vi "Read Waveform.vi"(8 "error in (no error)":errorcluster, 10 "Channel":T1, 11 "MSOX6004 in":refnum<class "MSOX6004.lvclass">) -> (0 "error out":errorcluster, 2 "Waveform":waveform(dbl)(graph), 3 "MSOX6004 out":refnum<class "MSOX6004.lvclass">)   [LabVIEW 2018, in "MSOX6004.lvlib" / "MSOX6004.lvclass"]
doc: "This Override method is used to initiate waveform acquisition. Select targeted channel at the 'Channel' control and output waveform data to the 'Waveform' indicator."
uses:
  MSOX6004.lvclass
  PPLs/Oscilloscope/Parent/Oscilloscope.lvlibp/Custom Controls/Analog Channels.ctl
  MSOX6004.lvclass/MSOX6004.ctl
  <instrlib>/Keysight InfiniiVision/Keysight InfiniiVision.lvlib
  PPLs/Oscilloscope/Parent/Oscilloscope.lvlibp
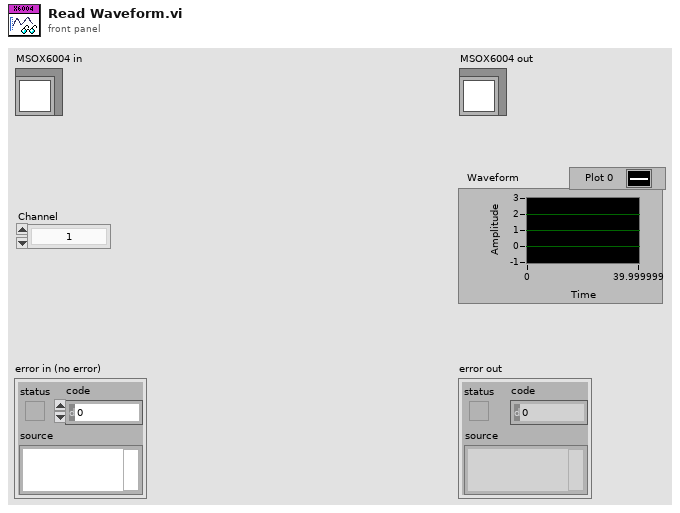
[diagram p1: front panel]
types:
  T1 = typedef "Oscilloscope.lvlibp/Analog Channels.ctl" = enum16{"1", "2", "3", "4", "5", "6", "7", "8", "9", "10", "11", "12", "13", "14", "15", "16"}
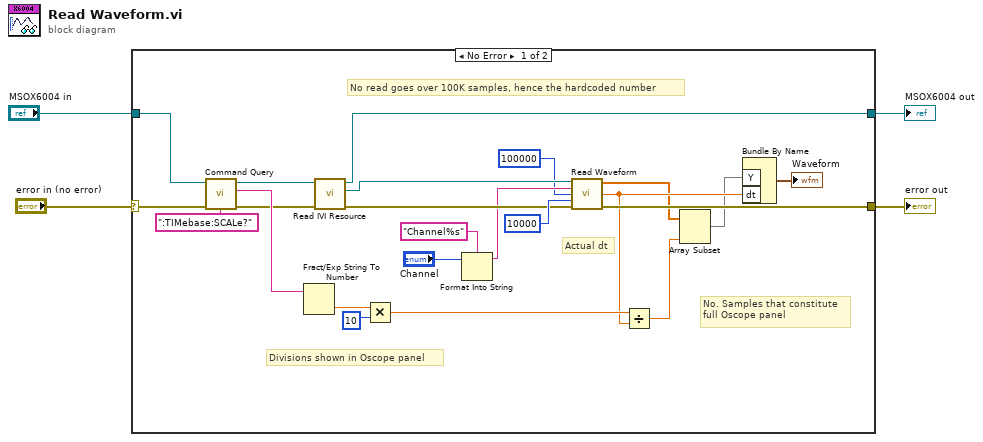
[diagram p0: block diagram]
diagram:
  n1 = case shown="No Error" "error in (no error)" {
    selector: "error in (no error)" -> [w22 w28]
    tunnel: "MSOX6004 in" -> [w23 w29]
    tunnel: [w16 w29] -> w2
    tunnel: [w15 w28] -> w1
    frame No Error {
      # "No. Samples that constitute\nfull Oscope panel"
      # "Actual dt"
      # "Divisions shown in Oscope panel"
      # "No read goes over 100K samples, hence the hardcoded number"
      n2 = call "Command Query.vi"("error in (no error)"=w22, "Command"=":TIMebase:SCALe?" ("channel name"), "MSOX6004 in"=w23) -> ("error out"=w6:errorcluster, "Response"=w20:string, "MSOX6004 out"=w7:refnum<class "MSOX6004.lvclass">)  [unwired: 6 in]
      n3 = Fract/Exp String To Number(string=w20) -> (number=w19:dbl)  [unwired: 3 in, 1 out]
      n4 = call "Read IVI Resource.vi"("error in (no error)"=w6, "MSOX6004 in"=w7) -> ("error out"=w17:errorcluster, "IVI Resource"=w13:refnum<k15>, "MSOX6004 out"=w16:refnum<class "MSOX6004.lvclass">)  [unwired: 7 in]
      n5 = Multiply(x=w19, y=u8 10) -> (x*y=w12:dbl)
      n6 = Format Into String(format string="Channel%s" ("channel name"), "Channel") -> (resulting string=w14:string)  [unwired: 2 in, 1 out]
      n7 = call <instrlib>:"Read Waveform.vi"("instrument handle"=w13, "channel name"=w14, "waveform size (2048)"=100000, "maximum time (0 ms)"=10000, "error in (no error)"=w17) -> ("x increment (s)"=w11:dbl, "waveform array (V)"=w10:dbl[], "error out"=w15:errorcluster)  [unwired: 5 in, 3 out]
      n8 = Divide(x=w12, y=w11) -> (x/y=w9:dbl)
      n9 = Array Subset(array=w10, length=w9) -> (w8:dbl[])  [unwired: 1 in]
      n10 = Bundle By Name("Y"=w8, "dt"=w11) -> (→"Waveform":waveform(dbl))  [unwired: 1 in]
    }
    frame Error {
    }
  }
  "error out" <- w1
  "MSOX6004 out" <- w2
